vi "10_кВ.vi"(0 "Вкл. РЗиА 2":bool, 2 "Вкл. РЗиА 1":bool, 7 "Time\ndelay":dbl) -> (1 "РЗиА  ВВОД 2":bool, 3 "РЗиА  ВВОД 1":bool, 8 "I 10 кВ ВВОД 2":i64(knob) scale=0.0..630.0, 9 "U 10 кВ ВВОД 2":i64(knob) caption="Вольтметр 10 кВ" scale=9000.0..11000.0, 10 "I 10 кВ ВВОД 1":i64(knob) scale=0.0..630.0, 11 "U 10 кВ ВВОД 1":i64(knob) caption="Вольтметр 10 кВ" scale=9000.0..11000.0)   [LabVIEW 2016]
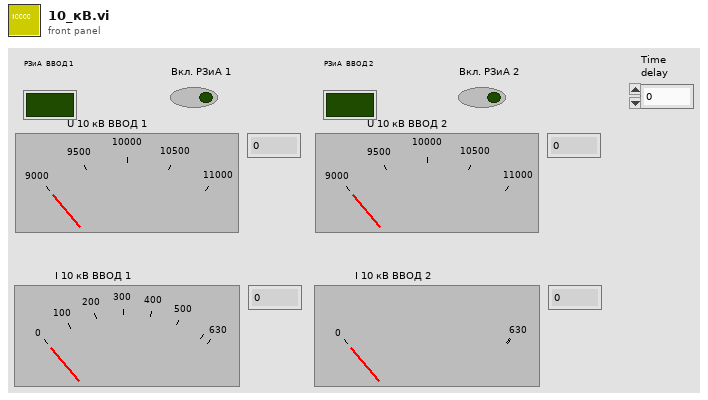
[diagram p1: front panel]
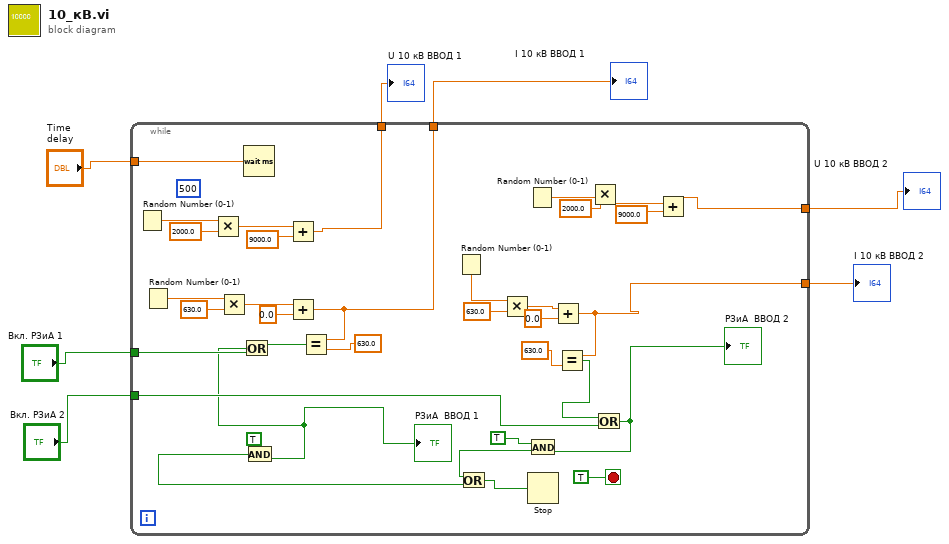
[diagram p0: block diagram]
diagram:
  n1 = while {
    tunnel: "Time\ndelay" -> [w16]
    tunnel: "Вкл. РЗиА 1" -> [w15]
    tunnel: "Вкл. РЗиА 2" -> [w14]
    tunnel: [w13] -> w4
    tunnel: [w12] -> w3
    tunnel: [w11] -> w2
    tunnel: [w10] -> w1
    stop <- TRUE stop-if-true
    (unwired) u32 500 ("milliseconds to wait")
    n2 = Random Number (0-1)() -> (number: 0 to 1=w42:dbl)
    n3 = Random Number (0-1)() -> (number: 0 to 1=w35:dbl)
    n4 = Multiply(x=w42, y=2000.0) -> (x*y=w40:dbl)
    n5 = Multiply(x=w35, y=630.0) -> (x*y=w37:dbl)
    n6 = Wait (ms)(milliseconds to wait=w16) -> ()  [unwired: 1 out]
    n7 = Add(x=w40, y=9000.0) -> (x+y=w13:dbl)
    n8 = Add(x=w37, y=0.0) -> (x+y=w12:dbl)
    n9 = Equal?(x=w12, y=630.0) -> (x = y?=w33:bool)
    n10 = Or(x=w33, y=w15) -> (x .or. y?=w8:bool)
    "РЗиА  ВВОД 1" <- w8
    n11 = And(x=TRUE, y=w8) -> (x .and. y?=w20:bool)
    n12 = Random Number (0-1)() -> (number: 0 to 1=w24:dbl)
    n13 = Multiply(x=w24, y=630.0) -> (x*y=w26:dbl)
    n14 = Random Number (0-1)() -> (number: 0 to 1=w31:dbl)
    n15 = Add(x=w26, y=0.0) -> (x+y=w10:dbl)
    n16 = Equal?(x=w10, y=630.0) -> (x = y?=w22:bool)
    n17 = Multiply(x=w31, y=2000.0) -> (x*y=w29:dbl)
    n18 = Or(x=w22, y=w14) -> (x .or. y?=w9:bool)
    "РЗиА  ВВОД 2" <- w9
    n19 = And(x=TRUE, y=w9) -> (x .and. y?=w19:bool)
    n20 = Or(x=w19, y=w20) -> (x .or. y?=w18:bool)
    n21 = Stop(stop? (T)=w18) -> ()
    n22 = Add(x=w29, y=9000.0) -> (x+y=w11:dbl)
  }
  "U 10 кВ ВВОД 1" <- w4
  "I 10 кВ ВВОД 1" <- w3
  "U 10 кВ ВВОД 2" <- w2
  "I 10 кВ ВВОД 2" <- w1
